vi "SetSweep_popup.vi"(2 "Input Line Command":string, 3 "error in (no error)":errorcluster) -> (8 "Cancel":bool, 9 "Output Line Command":string, 10 "error out":errorcluster)   [LabVIEW 2024]
uses:
  Device_List.ctl
  Unit_List.ctl
panel:
  in  "mode":T1 caption="Unit"
  in  "time":string="0" caption="Sweep time (min)"
  in  "Final":string="0" caption="Final Current (mA)"
  in  "platform":u16(ring) items=["Mac", "PC"]
  out "comment":string
  in  "Cancel Button":bool
  in  "OK Button":bool
  in  "VISA resource name":refnum<visa-resource-name>
  in  "Initial":string="0" caption="Initial Current (mA)"
  in  "Device":T2
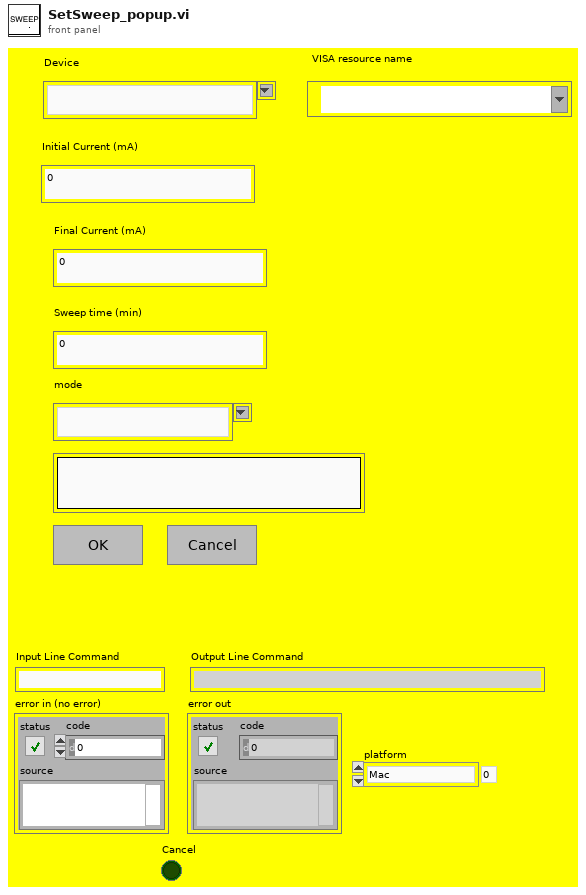
[diagram p1: front panel]
types:
  T1 = typedef "Unit_List.ctl" = string
  T2 = typedef "Device_List.ctl" = string
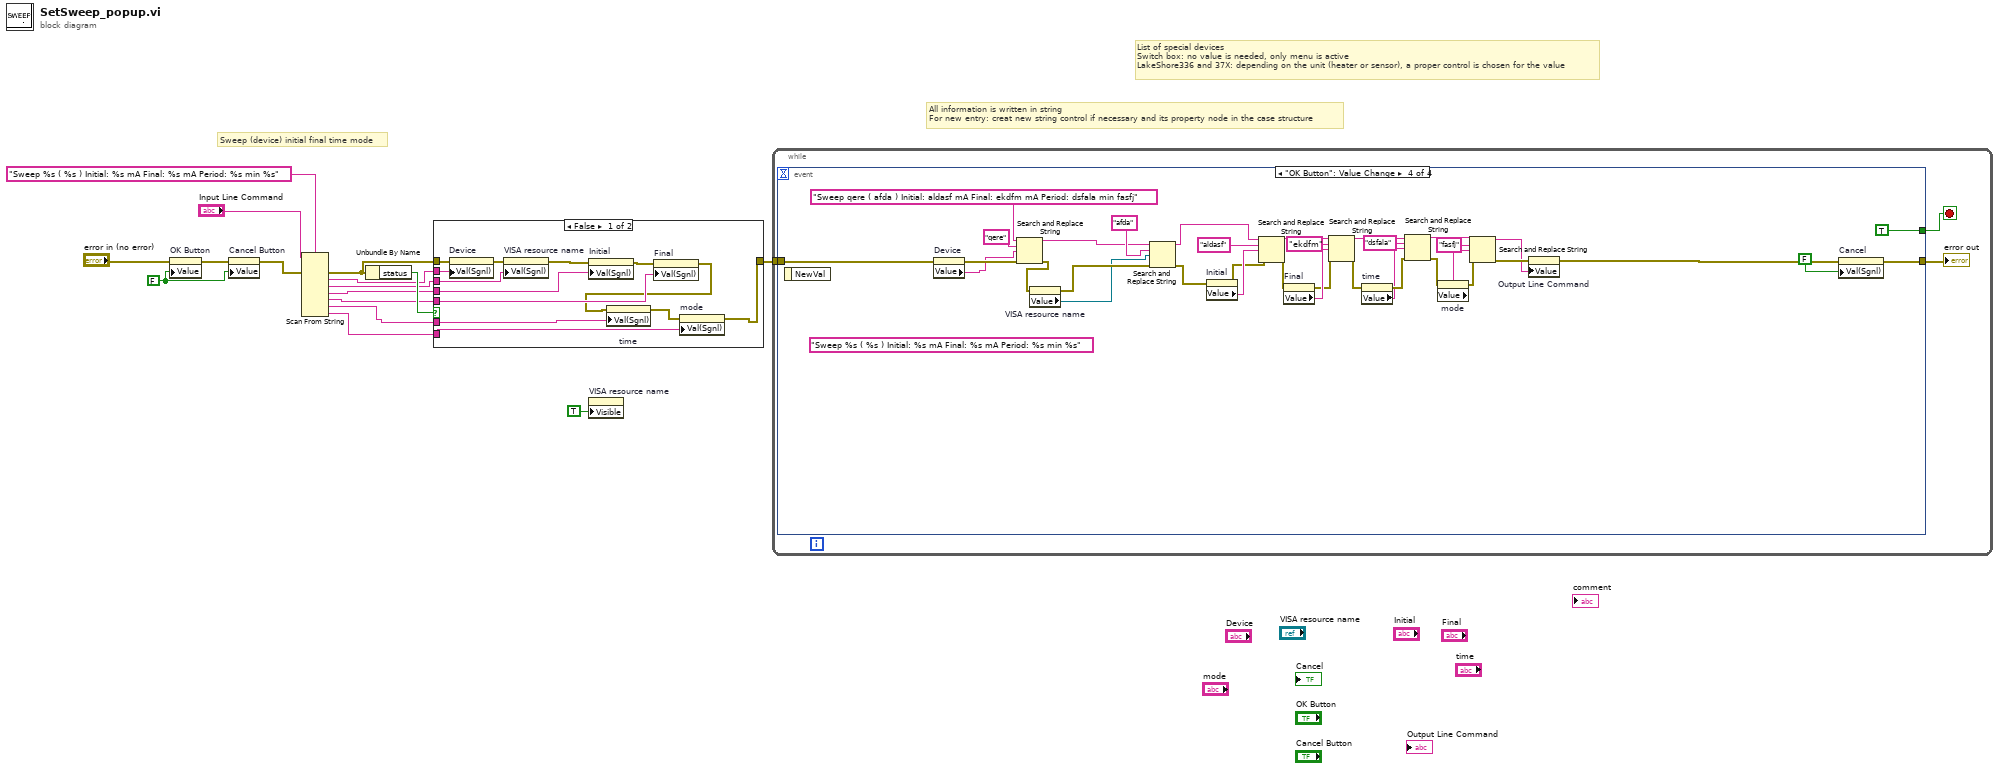
[diagram p0: block diagram]
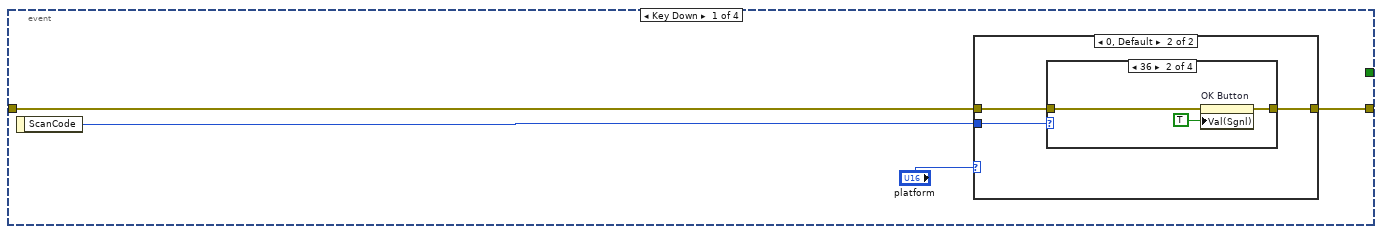
[diagram p2: hidden frame]
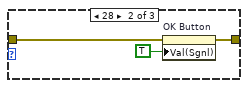
[diagram p4: hidden frame]
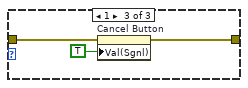
[diagram p5: hidden frame]
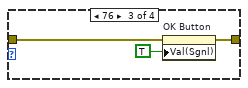
[diagram p7: hidden frame]
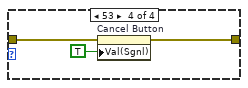
[diagram p8: hidden frame]
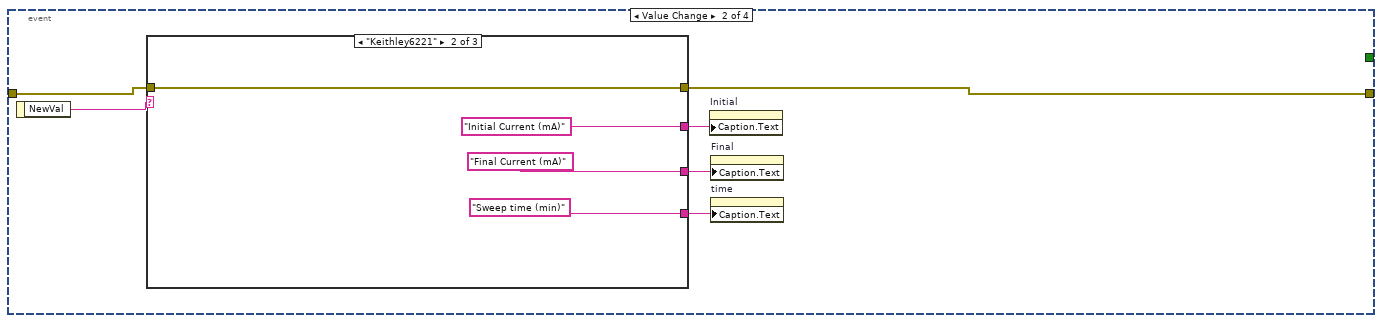
[diagram p9: hidden frame]
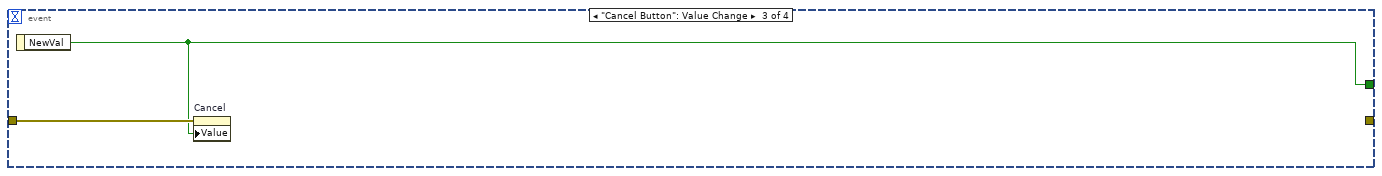
[diagram p12: hidden frame]
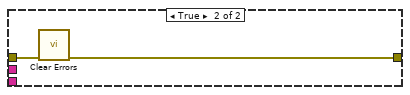
[diagram p13: hidden frame]
diagram:
  w14 = FALSE
  # "Sweep (device) initial final time mode"
  # "List of special devices\nSwitch box: no value is needed, only menu is active\nLakeShore336 and 37X: depending on the unit (heater or sensor), a proper control is chosen for the value"
  # "All information is written in string\nFor new entry: creat new string control if necessary and its property node in the case structure"
  n1 = property on="OK Button" class="Bool (strict)"(error in="error in (no error)", "Value"=w14) -> (error out=w15:errorcluster)  [unwired: 1 in, 1 out]
  n2 = property on="Cancel Button" class="Bool (strict)"(error in=w15, "Value"=w14) -> (error out=w13:errorcluster)  [unwired: 1 in, 1 out]
  n3 = Scan From String(format string="Sweep %s ( %s ) Initial: %s mA Final: %s mA Period: %s min %s", input string="Input Line Command", error in=w13) -> (error out=w9:errorcluster, output 1=w8:string, output 2=w7:string, output 3=w6:string, output 4=w5:string, output 5=w3:string, output 6=w2:string)  [unwired: 7 in, 2 out]
  n4 = Unbundle By Name(w9) -> ("status"=w10:bool)
  n5 = case shown="False" w10 {
    tunnel: w9 -> [w29 w31]
    tunnel: [w17 w30] -> w4
    tunnel: w8 -> [w28 _]
    tunnel: w7 -> [w26 _]
    tunnel: w6 -> [w24 _]
    tunnel: w5 -> [w22 _]
    tunnel: w3 -> [w21 _]
    tunnel: w2 -> [w18 _]
    frame False {
      n6 = property on="Device" class="CmbBox (strict)"(error in=w29, "Val(Sgnl)"=w28) -> (error out=w27:errorcluster)  [unwired: 1 in, 1 out]
      n7 = property on="VISA resource name" class="VISAName"(error in=w27, "Val(Sgnl)"=w26) -> (error out=w25:errorcluster)  [unwired: 1 in, 1 out]
      n8 = property on="Initial" class="Str"(error in=w25, "Val(Sgnl)"=w24) -> (error out=w23:errorcluster)  [unwired: 1 in, 1 out]
      n9 = property on="Final" class="Str"(error in=w23, "Val(Sgnl)"=w22) -> (error out=w20:errorcluster)  [unwired: 1 in, 1 out]
      n10 = property on="time" class="Str"(error in=w20, "Val(Sgnl)"=w21) -> (error out=w19:errorcluster)  [unwired: 1 in, 1 out]
      n11 = property on="mode" class="CmbBox (strict)"(error in=w19, "Val(Sgnl)"=w18) -> (error out=w17:errorcluster)  [unwired: 1 in, 1 out]
    }
    frame True {
      n12 = call <vilib>:"Clear Errors.vi"("error in (no error)"=w31) -> ("error out"=w30:errorcluster)  [unwired: 5 in, 1 out]
    }
  }
  n13 = property on="VISA resource name" class="VISAName"("Visible"=TRUE) -> ()  [unwired: 2 in, 2 out]
  n14 = while {
    tunnel: w4 -> [w34]
    stop <- w33 stop-if-true
    n15 = event shown="[3] \"OK Button\": Value Change" {
      selector: _ -> [_ _ _ _]
      dyn-events: _ -> [_ _ _ _]
      timeout: _ -> [_ _ _ _]
      tunnel: w34 -> [w37 w65 w75 w109]
      tunnel: [_ _ w74 TRUE ("NewVal")] -> w33
      tunnel: [w36 w67 _ w96] -> w32
      event Key Down {
        n16 = event-data() -> ("ScanCode"=w38:i16)  [unwired: 1 in]
        n17 = case shown="0, Default" "platform" {
          tunnel: w38 -> [w41 w51]
          tunnel: w37 -> [w40 w50]
          tunnel: [w39 w49] -> w36
          frame 1 {
            n18 = case shown="Default" w41 {
              tunnel: w40 -> [w42 w45 w48]
              tunnel: [w42 w43 w46] -> w39
              frame Default {
              }
              frame 28 {
                n19 = property on="OK Button" class="Bool (strict)"(error in=w45, "Val(Sgnl)"=TRUE) -> (error out=w43:errorcluster)  [unwired: 1 in, 1 out]
              }
              frame 1 {
                n20 = property on="Cancel Button" class="Bool (strict)"(error in=w48, "Val(Sgnl)"=TRUE ("Value (Signaling)")) -> (error out=w46:errorcluster)  [unwired: 1 in, 1 out]
              }
            }
          }
          frame 0, Default {
            n21 = case shown="36" w51 {
              tunnel: w50 -> [w52 w55 w58 w61]
              tunnel: [w52 w53 w56 w59] -> w49
              frame Default {
              }
              frame 36 {
                n22 = property on="OK Button" class="Bool (strict)"(error in=w55, "Val(Sgnl)"=TRUE) -> (error out=w53:errorcluster)  [unwired: 1 in, 1 out]
              }
              frame 76 {
                n23 = property on="OK Button" class="Bool (strict)"(error in=w58, "Val(Sgnl)"=TRUE) -> (error out=w56:errorcluster)  [unwired: 1 in, 1 out]
              }
              frame 53 {
                n24 = property on="Cancel Button" class="Bool (strict)"(error in=w61, "Val(Sgnl)"=TRUE ("Value (Signaling)")) -> (error out=w59:errorcluster)  [unwired: 1 in, 1 out]
              }
            }
          }
        }
      }
      event Value Change {
        n25 = event-data() -> ("NewVal"=w66:T2)  [unwired: 1 in]
        n26 = case shown="\"Keithley6221\"" w66 {
          tunnel: w65 -> [w68 w72 w73]
          tunnel: [w68 w72 w73] -> w67
          tunnel: [_ "Initial Current (mA)" ("Caption.Text") _] -> w64
          tunnel: [_ "Final Current (mA)" ("Caption.Text") _] -> w63
          tunnel: [_ "Sweep time (min)" ("Caption.Text") _] -> w62
          frame "False", Default {
          }
          frame "Keithley6221" {
          }
          frame "Generic device" {
          }
        }
        n27 = property on="Initial" class="Str"("Caption.Text"=w64) -> ()  [unwired: 2 in, 2 out]
        n28 = property on="Final" class="Str"("Caption.Text"=w63) -> ()  [unwired: 2 in, 2 out]
        n29 = property on="time" class="Str"("Caption.Text"=w62) -> ()  [unwired: 2 in, 2 out]
      }
      event "Cancel Button": Value Change {
        n30 = event-data() -> ("NewVal"=w74:bool)  [unwired: 1 in]
        n31 = property on="Cancel" class="Bool (strict)"(error in=w75, "Value"=w74) -> ()  [unwired: 1 in, 2 out]
      }
      event "OK Button": Value Change {
        (unwired) "Sweep %s ( %s ) Initial: %s mA Final: %s mA Period: %s min %s" ("format string")
        n32 = event-data() -> ()  [unwired: 1 in, 1 out]
        n33 = property on="Device" class="CmbBox (strict)"(error in=w109) -> (error out=w108:errorcluster, "Value"=w94:T2)  [unwired: 1 in, 1 out]
        n34 = Search and Replace String(input string="Sweep qere ( afda ) Initial: aldasf mA Final: ekdfm mA Period: dsfala min fasfj", search string="qere", replace string=w94, error in=w108) -> (result string=w106:string, error out=w93:errorcluster)  [unwired: 4 in, 2 out]
        n35 = property on="VISA resource name" class="VISAName"(error in=w93) -> (error out=w92:errorcluster, "Value"=w91:refnum<visa-resource-name>)  [unwired: 1 in, 1 out]
        n36 = Search and Replace String(input string=w106, search string="afda", replace string=w91, error in=w92) -> (result string=w105:string, error out=w102:errorcluster)  [unwired: 4 in, 2 out]
        n37 = property on="Initial" class="Str"(error in=w102) -> (error out=w101:errorcluster, "Value"=w103:string)  [unwired: 1 in, 1 out]
        n38 = Search and Replace String(input string=w105, search string="aldasf", replace string=w103, error in=w101) -> (result string=w90:string, error out=w88:errorcluster)  [unwired: 4 in, 2 out]
        n39 = property on="Final" class="Str"(error in=w88) -> (error out=w87:errorcluster, "Value"=w89:string)  [unwired: 1 in, 1 out]
        n40 = Search and Replace String(input string=w90, search string="ekdfm", replace string=w89, error in=w87) -> (result string=w80:string, error out=w81:errorcluster)  [unwired: 4 in, 2 out]
        n41 = property on="time" class="Str"(error in=w81) -> (error out=w86:errorcluster, "Value"=w82:string)  [unwired: 1 in, 1 out]
        n42 = Search and Replace String(input string=w80, search string="dsfala", replace string=w82, error in=w86) -> (result string=w79:string, error out=w78:errorcluster)  [unwired: 4 in, 2 out]
        n43 = property on="mode" class="CmbBox (strict)"(error in=w78) -> (error out=w77:errorcluster, "Value"=w76:T1)  [unwired: 1 in, 1 out]
        n44 = Search and Replace String(input string=w79, search string="fasfj", replace string=w76, error in=w77) -> (result string=w99:string, error out=w100:errorcluster)  [unwired: 4 in, 2 out]
        n45 = property on="Output Line Command" class="Str"(error in=w100, "Value"=w99) -> (error out=w98:errorcluster)  [unwired: 1 in, 1 out]
        n46 = property on="Cancel" class="Bool (strict)"(error in=w98, "Val(Sgnl)"=FALSE ("Cancel")) -> (error out=w96:errorcluster)  [unwired: 1 in, 1 out]
      }
    }
    "error out" <- w32
  }
